vi "Funcion h 15.vi"(10 "y":u16, 11 "x":u16) -> (2 "y(t+1)":u16, 3 "x(t+1)":u16)   [LabVIEW 2023]
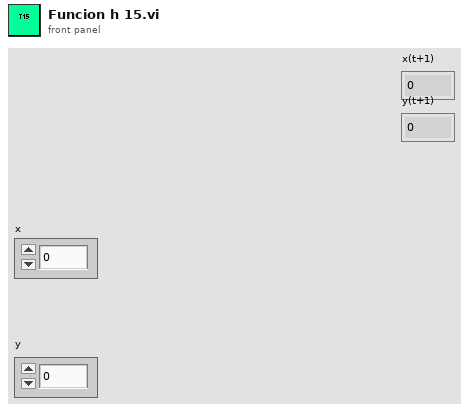
[diagram p1: front panel]
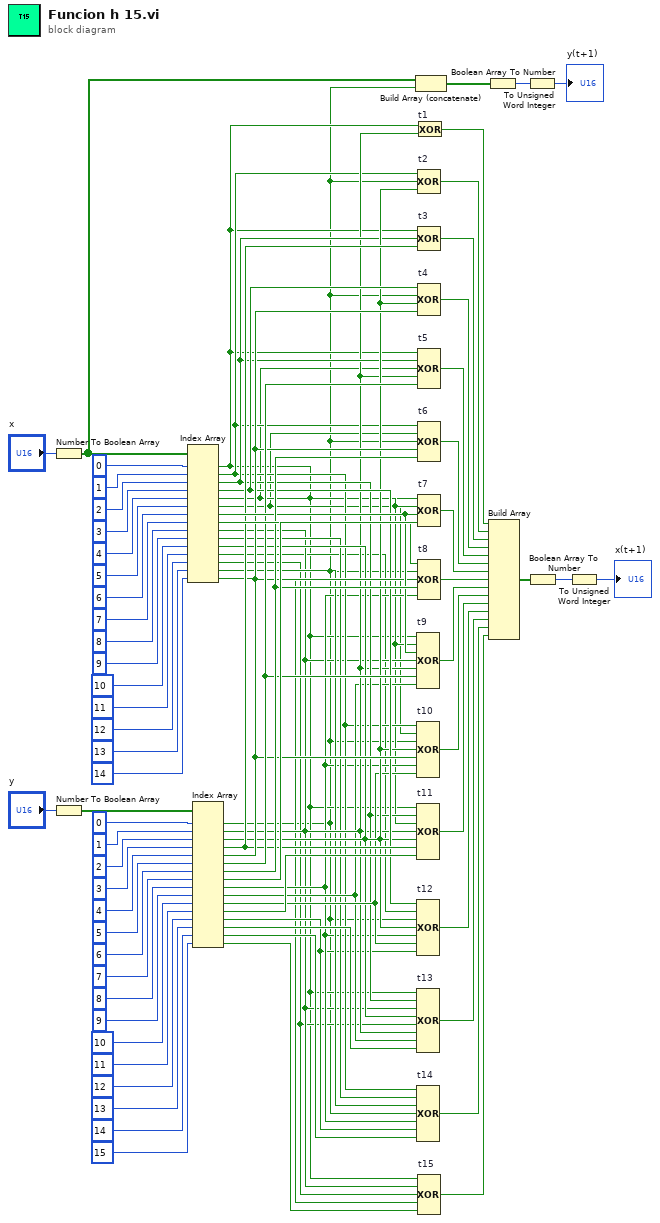
[diagram p0: block diagram]
diagram:
  n1 = Number To Boolean Array(number="x") -> (Boolean array=w8:bool[])
  n2 = Number To Boolean Array(number="y") -> (Boolean array=w54:bool[])
  n3 = Index Array(array=w8, index #1=0 ("index"), index #2=1 ("index"), index #3=2 ("index"), index #4=3 ("index"), index #5=4 ("index"), index #6=5 ("index"), index #7=6 ("index"), index #8=7 ("index"), index #9=8 ("index"), index #10=9 ("index"), index #11=10 ("index"), index #12=11 ("index"), index #13=12 ("index"), index #14=13 ("index"), index #15=14 ("index")) -> (element #1=w7:bool, element #2=w24:bool, element #3=w30:bool, element #4=w34:bool, element #5=w12:bool, element #6=w11:bool, element #7=w43:bool, element #8=w45:bool, element #9=w17:bool, element #10=w23:bool, element #11=w29:bool, element #12=w10:bool, element #13=w16:bool, element #14=w22:bool, element #15=w15:bool)
  n4 = Index Array(array=w54, index #1=0 ("index"), index #2=1 ("index"), index #3=2 ("index"), index #4=3 ("index"), index #5=4 ("index"), index #6=5 ("index"), index #7=6 ("index"), index #8=7 ("index"), index #9=8 ("index"), index #10=9 ("index"), index #11=10 ("index"), index #12=11 ("index"), index #13=12 ("index"), index #14=13 ("index"), index #15=14 ("index"), index #16=15 ("index")) -> (element #1=w6:bool, element #2=w28:bool, element #3=w33:bool, element #4=w38:bool, element #5=w39:bool, element #6=w42:bool, element #7=w44:bool, element #8=w47:bool, element #9=w21:bool, element #10=w27:bool, element #11=w32:bool, element #12=w37:bool, element #13=w20:bool, element #14=w26:bool, element #15=w19:bool, element #16=w14:bool)
  n5 = Exclusive Or "t1"(1:w28, 2:w7) -> (0:w52:bool)
  n6 = Build Array (concatenate)(w8, w6) -> (w5:bool[])
  n7 = Compound Arithmetic op=XOR "t9"(w7, w12, w43, w17, w28, w42, w27) -> (w40:bool)
  n8 = Compound Arithmetic op=XOR "t10"(w24, w11, w6, w33, w39, w21, w32) -> (w36:bool)
  n9 = Compound Arithmetic op=XOR "t11"(w7, w30, w12, w17, w29, w38, w37) -> (w35:bool)
  n10 = Compound Arithmetic op=XOR "t12"(w34, w10, w6, w33, w21, w32, w20) -> (w31:bool)
  n11 = Compound Arithmetic op=XOR "t13"(w7, w30, w17, w29, w16, w28, w27, w26) -> (w25:bool)
  n12 = Compound Arithmetic op=XOR "t14"(w24, w23, w22, w6, w21, w20, w19) -> (w18:bool)
  n13 = Compound Arithmetic op=XOR "t2"(w24, w6, w33) -> (w53:bool)
  n14 = Compound Arithmetic op=XOR "t3"(w7, w30, w38) -> (w51:bool)
  n15 = Compound Arithmetic op=XOR "t4"(w34, w6, w33, w39) -> (w50:bool)
  n16 = Compound Arithmetic op=XOR "t5"(w7, w30, w12, w28, w42) -> (w49:bool)
  n17 = Compound Arithmetic op=XOR "t6"(w24, w11, w6, w39, w44) -> (w48:bool)
  n18 = Compound Arithmetic op=XOR "t7"(w7, w12, w43, w47) -> (w46:bool)
  n19 = Compound Arithmetic op=XOR "t8"(w45, w6, w39, w44, w21) -> (w41:bool)
  n20 = Compound Arithmetic op=XOR "t15"(w7, w17, w16, w15, w14) -> (w13:bool)
  n21 = Boolean Array To Number(Boolean array=w5) -> (number=w4:u32)
  n22 = Build Array(w52, w53, w51, w50, w49, w48, w46, w41, w40, w36, w35, w31, w25, w18, w13) -> (w9:bool[])
  n23 = To Unsigned Word Integer(number=w4) -> (unsigned 16bit integer=→"y(t+1)":u16)
  n24 = Boolean Array To Number(Boolean array=w9) -> (number=w2:u32)
  n25 = To Unsigned Word Integer(number=w2) -> (unsigned 16bit integer=→"x(t+1)":u16)
